vi "Touch_Sensor_EV3.vi"() -> ()   [LabVIEW 2012]
uses:
  SubVIs/LVPresent_Globals.vi
panel:
  in  "Tab Control":enum32{"Page 1", "Page 2"}(tab)
  in  "Open":bool
  in  "Need a hint":bool
  in  "Back":bool
  in  "Ans. 4":bool
  in  "Ans. 5":bool
  in  "Ans. 6":bool
  # "Touch Sensor (and more!)\n\nLet's test out the touch sensor! First, attach the touch sensor onto the robot. Then, write some code so that the robot stops before it drives off the edge of a table. Click the Open button to start a new VI. If you're stuck on how to add the sensor, check out the EV3 manual  or just experiment with legos!"
  # "Step 2:\n\nAfter you get the code running, try enhancing your code so that the robot backs up and then rotates (any amount) after it reaches the edge."
  # "Extra Challenge:\n\nNow, enable the robot to repeat this process until the robot spots a red object on the table, and then have the robot stop 5 cm in front of the object (you will need multiple sensors for this)."
  # "Hint 1: Think about how you can get the touch sensor to react when the robot is on the table, compared to when it is driving off the table. \n\n\n\n\n\nHint 2:  In order to have the robot turn, think about what ports you should use. Also, feel free to make the robot rotate a set amount each time, or a variable amount. \n\n\n\n\n\nHint 3: Think about where to use each sensor, in order to get it to perform the function you want it to do at a given time."
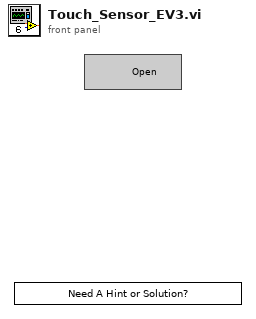
[diagram p1: front panel]
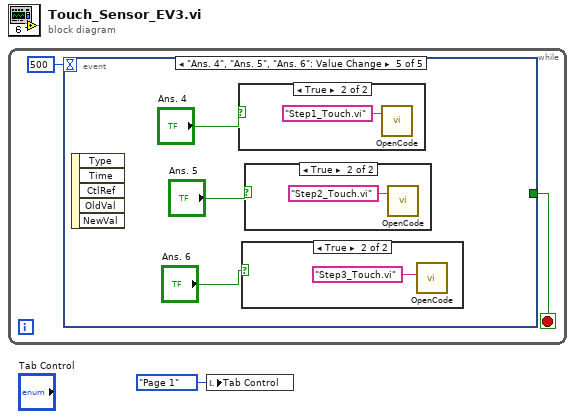
[diagram p0: block diagram]
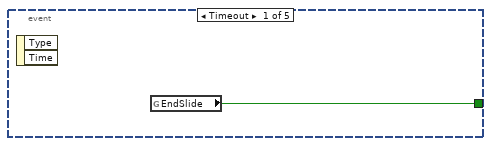
[diagram p2: hidden frame]
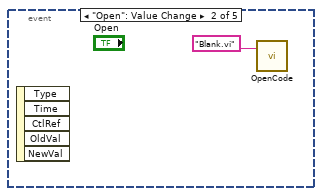
[diagram p3: hidden frame]
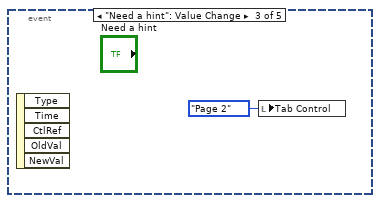
[diagram p4: hidden frame]
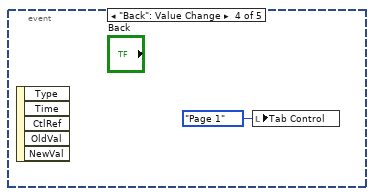
[diagram p5: hidden frame]
diagram:
  n1 = while {
    stop <- w3 stop-if-true
    n2 = event shown="[4] \"Ans. 4\", \"Ans. 5\", \"Ans. 6\": Value Change" {
      selector: _ -> [_ _ _ _ _]
      dyn-events: _ -> [_ _ _ _ _]
      timeout: 500 -> [_ _ _ _ _]
      tunnel: [w4 _ _ _ _] -> w3
      event Timeout {
        n3 = event-data() -> ()  [unwired: 1 in, 2 out]
        n4 = global read "LVPresent_Globals.vi" "EndSlide"() -> (w4:bool)
      }
      event "Open": Value Change {
        n5 = event-data() -> ()  [unwired: 1 in, 5 out]
        n6 = call "OpenCode.vi"("Code name"="Blank.vi") -> ()  [unwired: 3 in]
      }
      event "Need a hint": Value Change {
        n7 = event-data() -> ()  [unwired: 1 in, 5 out]
        n8 = local write "Tab Control"(enum32{"Page 1", "Page 2"}."Page 2" ("Tab Control")) -> ()
      }
      event "Back": Value Change {
        n9 = event-data() -> ()  [unwired: 1 in, 5 out]
        n10 = local write "Tab Control"(enum32{"Page 1", "Page 2"}."Page 1" ("Tab Control")) -> ()
      }
      event "Ans. 4", "Ans. 5", "Ans. 6": Value Change {
        n11 = event-data() -> ()  [unwired: 1 in, 5 out]
        n12 = case shown="True" "Ans. 4" {
          frame False {
          }
          frame True {
            n13 = call "OpenCode.vi"("Code name"="Step1_Touch.vi") -> ()  [unwired: 3 in]
          }
        }
        n14 = case shown="True" "Ans. 6" {
          frame False {
          }
          frame True {
            n15 = call "OpenCode.vi"("Code name"="Step3_Touch.vi") -> ()  [unwired: 3 in]
          }
        }
        n16 = case shown="True" "Ans. 5" {
          frame False {
          }
          frame True {
            n17 = call "OpenCode.vi"("Code name"="Step2_Touch.vi") -> ()  [unwired: 3 in]
          }
        }
      }
    }
  }
  n18 = local write "Tab Control"(enum32{"Page 1", "Page 2"}."Page 1" ("Tab Control")) -> ()
